vi "final.vi"() -> ()   [LabVIEW 2013]
panel:
  out "keyboard_now":T1
  in  "command":T2
  out "current_command":T2
  in  "R_ip":bool
  out "test":bool
  in  "WR":T3
  out "Flags":T4
  in  "-":bool
  out "output":T5
  in  "tick":bool
  in  "clear all":bool
  in  "keys":T6
  # "A - 10000\nB - 10001\n\nax - 00100\nbx - 00101\ncx - 00110\ndx - 00111\n\nio - 01000"
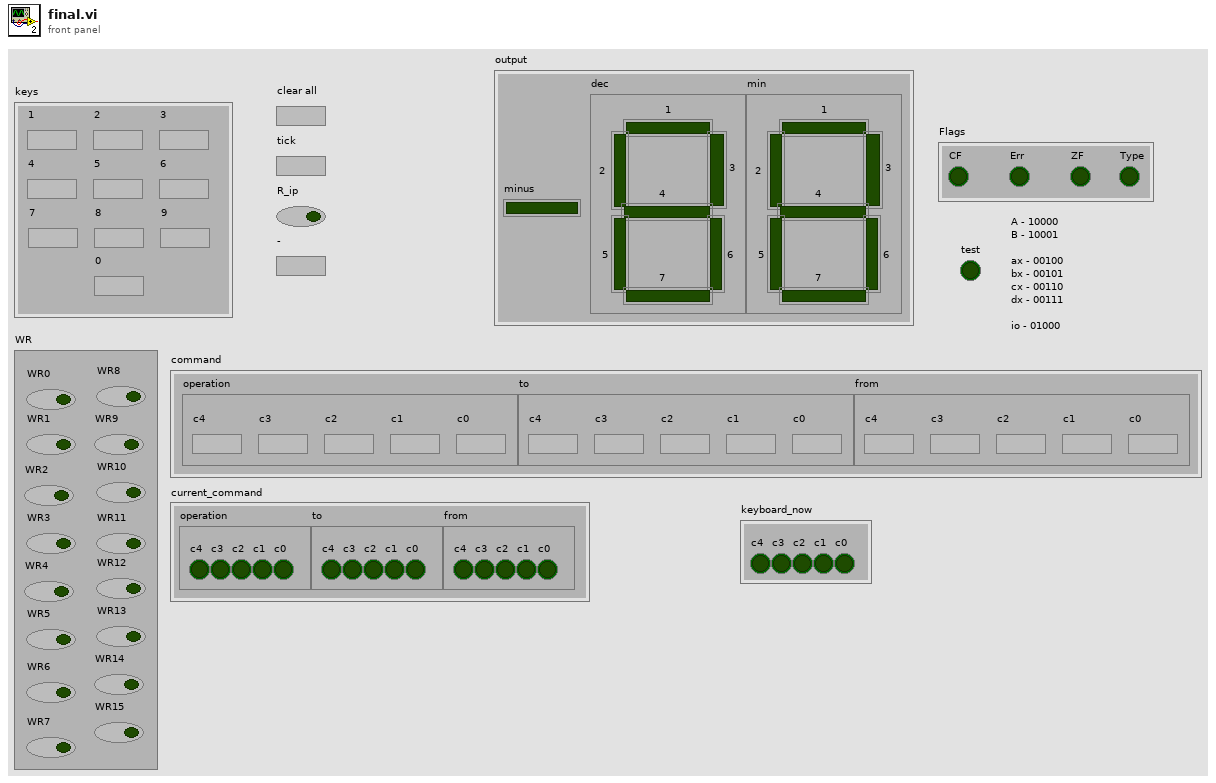
[diagram p1: front panel]
types:
  T1 = cluster{"c4":bool, "c3":bool, "c2":bool, "c1":bool, "c0":bool}
  T2 = cluster{"operation":cluster{"c4":bool, "c3":bool, "c2":bool, "c1":bool, "c0":bool}, "to":cluster{"c4":bool, "c3":bool, "c2":bool, "c1":bool, "c0":bool}, "from":cluster{"c4":bool, "c3":bool, "c2":bool, "c1":bool, "c0":bool}}
  T3 = cluster{"WR0":bool, "WR1":bool, "WR2":bool, "WR3":bool, "WR4":bool, "WR5":bool, "WR6":bool, "WR7":bool, "WR8":bool, "WR9":bool, "WR10":bool, "WR11":bool, "WR12":bool, "WR13":bool, "WR14":bool, "WR15":bool}
  T4 = cluster{"CF":bool, "Err":bool, "ZF":bool, "Type":bool}
  T5 = cluster{"minus":bool, "dec":cluster{"1":bool, "2":bool, "3":bool, "4":bool, "5":bool, "6":bool, "7":bool}, "min":cluster{"1":bool, "2":bool, "3":bool, "4":bool, "5":bool, "6":bool, "7":bool}}
  T6 = cluster{"1":bool, "2":bool, "3":bool, "4":bool, "5":bool, "6":bool, "7":bool, "8":bool, "9":bool, "0":bool}
  T7 = cluster{"x4":bool, "x3":bool, "x2":bool, "x1":bool, "x0":bool}
  T8 = cluster{"command_out":cluster{"c4":bool, "c3":bool, "c2":bool, "c1":bool, "c0":bool}, "to_out":cluster{"c4":bool, "c3":bool, "c2":bool, "c1":bool, "c0":bool}, "from_out":cluster{"c4":bool, "c3":bool, "c2":bool, "c1":bool, "c0":bool}}
  T9 = cluster{"RD":cluster{"ax":bool, "bx":bool, "cx":bool, "dx":bool}, "wr":cluster{"ax":bool, "bx":bool, "cx":bool, "dx":bool}}
  T10 = cluster{"a_flags":cluster{"rd":bool, "wr":bool}, "b_flags":cluster{"rd":bool, "wr":bool}}
  T11 = cluster{"R4":bool, "R3":bool, "R2":bool, bool, "R0":bool}
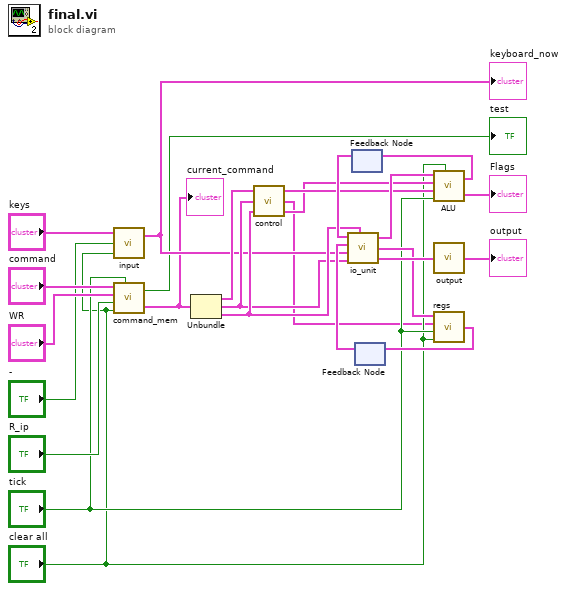
[diagram p0: block diagram]
diagram:
  n1 = call "input.vi"("r"="clear all", "-"="-", "keys"="keys") -> ("output"=w6:T7)  [unwired: 1 out]
  "keyboard_now" <- w6
  n2 = call "command_mem.vi"("input"="command", "WR"="WR", "R_ip"="R_ip", "R"="clear all", "С"="tick") -> ("test"=→"test":bool, "output"=w5:T8)
  "current_command" <- w5
  n3 = Unbundle(w5) -> ("command_out"=w8:T1, "to_out"=w10:T1, "from_out"=w11:T1)
  n4 = call "control.vi"("from"=w11, "to"=w10, "operation_code"=w8) -> ("operation"=w7:T1, "regs_control"=w1:T9, "alu_regs_control"=w9:T10)
  n5 = feedback #1() -> (w18:T11)  [unwired: 1 in]
  n6 = feedback #2() -> (w21:T1)  [unwired: 1 in]
  n7 = call "io_unit.vi"("from_alu"=w18, "from_regs"=w21, "from_input"=w6, "to"=w10, "from"=w11) -> ("to_alu"=w20:T7, "to_regs"=w23:T7, "to_output"=w24:T7)
  n8 = call "ALU.vi"("A"=w20, "Control"=w7, "alu_regs_flags"=w9, "tick"="tick", "clear all"="clear all") -> ("acc_content"=w19:T11, "Flags"=→"Flags":T4)
  n9 = feedback-in #1(w19) -> ()
  n10 = call "output.vi"("input"=w24) -> ("output"=→"output":T5)
  n11 = call "regs.vi"("clear all"="clear all", "tick"="tick", "regs_flags"=w1, "input"=w23) -> ("output"=w22:T1)
  n12 = feedback-in #2(w22) -> ()
